vi "SignalReceiver.GetSetpoint.vi"(8 "error in (no error)":errorcluster, 11 "SignalReceiver":refnum<class "SignalReceiver.lvclass">) -> (0 "error out":errorcluster, 2 "Setpoint":dbl, 3 "SignalReceiver out":refnum<class "SignalReceiver.lvclass">)   [LabVIEW 2020, in "ECU_Diagnose.lvlib" / "SignalReceiver.lvclass"]
doc: "---------------------------------------------------------------\nJKI State Machine Objects™\nhttp://jki.net/state-machine-objects/\nCopyright (C) 2005-2015, JKI <info@jki.net>\nALL RIGHTS RESERVEDJKI State Machine Objects (SMO) 1.0.0.5\nJKI - JKI\nCopyright (c) 2016, JKI"
uses:
  SignalReceiver.lvclass
panel:
  # "For instructions on how to use the JKI State Machine Objects, examples and video tutorials, visit:\nhttp://jki.net/state-machine-objects/\n\nJKI State Machine Objects™\nhttp://jki.net/state-machine-objects/\nCopyright (C) 2005-2015, JKI <info@jki.net>\nALL RIGHTS RESERVED"
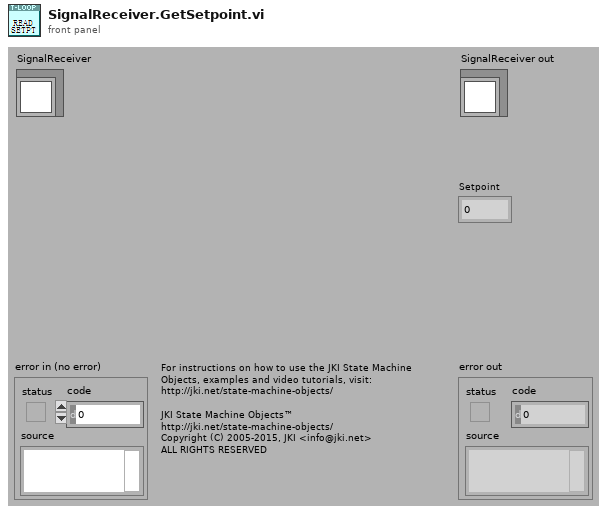
[diagram p1: front panel]
types:
  T1 = typedef "ECU_Diagnose.lvlib/SignalReceiver.lvclass/PrivateData--Ref.ctl" = refnum<data-value>
  T2 = typedef "ECU_Diagnose.lvlib/SignalReceiver.lvclass/PrivateData--Cluster.ctl" = cluster{"Public Events":T3, "Private Events":T4, "SignalArrySelect":T5, "SignalDataReciArry":T6}
  T3 = typedef "ECU_Diagnose.lvlib/SignalReceiver.lvclass/PublicEvents--Cluster.ctl" = cluster{"Setpoint Changed":refnum<user-event>, "Value Changed":refnum<user-event>}
  T4 = typedef "ECU_Diagnose.lvlib/SignalReceiver.lvclass/PrivateEvents--Cluster.ctl" = cluster{"AsyncMethod":refnum<user-event>, "Start_Stop":refnum<user-event>}
  T5 = typedef "ECU_Diagnose.lvlib/SignalReceiver.lvclass/SignalArrySelecte.ctl" = cluster{"Port_No.":refnum<k21>, "XNET Signal":refnum<k21>[]}
  T6 = typedef "ECU_Diagnose.lvlib/SignalReceiver.lvclass/SignalDataArry.ctl" = cluster{"SignalDataReceiveArry":dbl[][], "Update":bool}
  T7 = typedef "SignalReceiver.lvclass/Data.ctl" = dbl
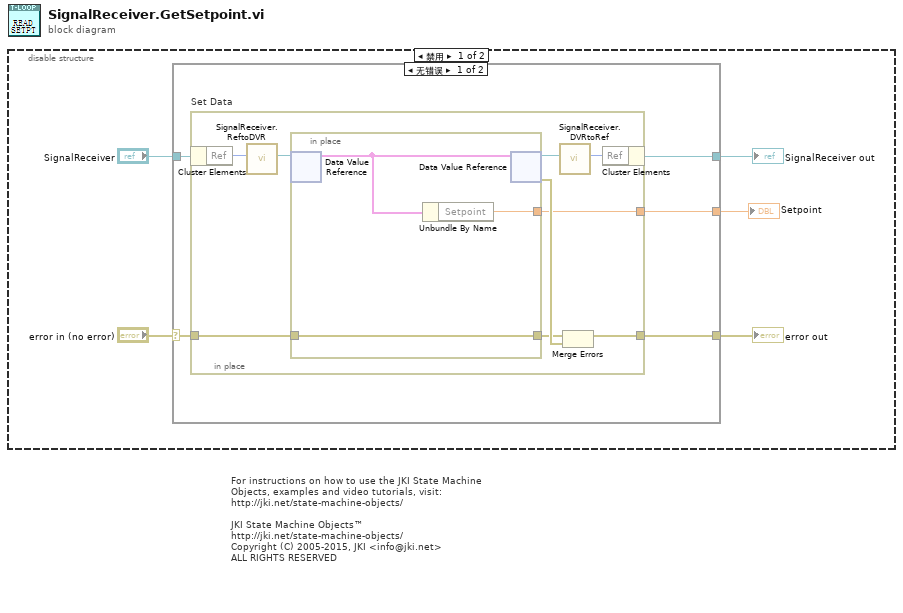
[diagram p0: block diagram]
diagram:
  # "For instructions on how to use the JKI State Machine Objects, examples and video tutorials, visit:\nhttp://jki.net/state-machine-objects/\n\nJKI State Machine Objects™\nhttp://jki.net/state-machine-objects/\nCopyright (C) 2005-2015, JKI <info@jki.net>\nALL RIGHTS RESERVED"
  n1 = disable-structure shown="禁用" {
    frame Disabled {
      n2 = case shown="无错误" "error in (no error)" {
        selector: "error in (no error)" -> [w9 w23]
        tunnel: "SignalReceiver" -> [w10 w24]
        tunnel: [w8 w23] -> w4
        tunnel: [w7 w24] -> w3
        tunnel: [w6 _] -> w1
        frame No Error {
          n3 = in-place "Set Data" {
            in-place-border: w9 -> [w19]
            in-place-border: [w16] -> w8
            in-place-border: [w11] -> w6
            n4 = in-place-cluster #1(w10) -> ("Ref"=w15:u32)
            n5 = call "SignalReceiver.ReftoDVR.vi"("Ref"=w15) -> ("Ref"=w14:T1)  [unwired: 10 in]
            n6 = in-place {
              in-place-border: w19 -> [w22]
              in-place-border: [w22] -> w17
              in-place-border: [w21] -> w11
              n7 = in-place-dvr #2(w14) -> (w20:T2)  [unwired: 1 out]
              n8 = Unbundle By Name(w20) -> ("Setpoint"=w21:T7)
              n9 = in-place-dvr #2(w20) -> (w13:T1, w18:errorcluster)
            }
            n10 = call "SignalReceiver.DVRtoRef.vi"("Ref"=w13) -> ("Ref"=w12:u32)  [unwired: 10 in]
            n11 = Merge Errors(w17, w18) -> (w16:errorcluster)
            n12 = in-place-cluster #1("Ref"=w12) -> (w7:refnum<class "SignalReceiver.lvclass">)
          }
        }
        frame Error {
        }
      }
      "error out" <- w4
      "SignalReceiver out" <- w3
      "Setpoint" <- w1
    }
    frame Enabled {
    }
  }
